vi "execute.vi"(8 "error in (no error)":errorcluster, 9 "ParameterString":string, 10 "ObjectCluster":T1, 11 "AirConditionCommand in":refnum<class "AirConditionCommand.lvclass">) -> (0 "error out":errorcluster, 2 "ObjectCluster Out":T1, 3 "AirConditionCommand out":refnum<class "AirConditionCommand.lvclass">)   [LabVIEW 2013, in "AirConditionCommand.lvclass"]
uses:
  AirConditionCommand.lvclass
  Command.lvclass/ObjectCluster.ctl
  AirCondition.lvclass/AirCondition.lvclass
  RoomLight.lvclass/RoomLight.lvclass
  OutDoorLight.lvclass/OutDoorLight.lvclass
  Television.lvclass/Television.lvclass
  Stereo.lvclass/Stereo.lvclass
  Command.lvclass/Command.lvclass
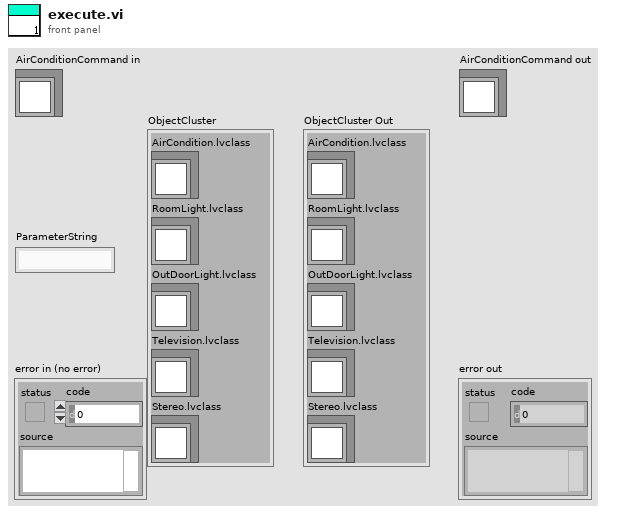
[diagram p1: front panel]
types:
  T1 = typedef "Command.lvclass/ObjectCluster.ctl" = cluster{"AirCondition.lvclass":refnum<class "AirCondition.lvclass">, "RoomLight.lvclass":refnum<class "RoomLight.lvclass">, "OutDoorLight.lvclass":refnum<class "OutDoorLight.lvclass">, "Television.lvclass":refnum<class "Television.lvclass">, "Stereo.lvclass":refnum<class "Stereo.lvclass">}
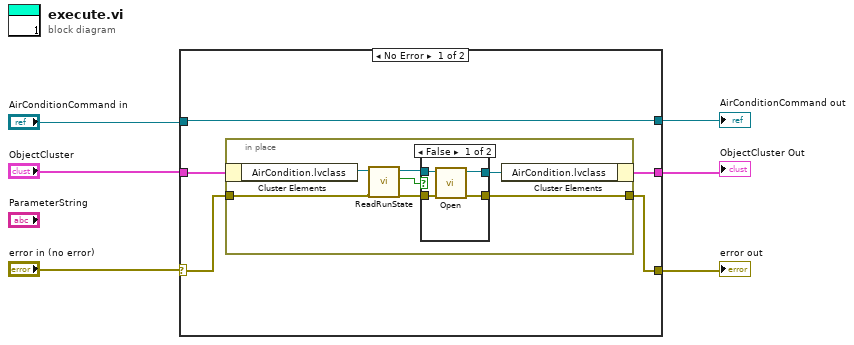
[diagram p0: block diagram]
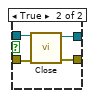
[diagram p2: hidden frame]
diagram:
  n1 = case shown="No Error" "error in (no error)" {
    selector: "error in (no error)" -> [w10 w27]
    tunnel: "ObjectCluster" -> [w11 w28]
    tunnel: "AirConditionCommand in" -> [w7 w29]
    tunnel: [w9 w27] -> w2
    tunnel: [w8 w28] -> w1
    tunnel: [w7 w29] -> w5
    frame No Error {
      n2 = in-place {
        in-place-border: w10 -> [w15]
        in-place-border: [w17] -> w9
        n3 = in-place-cluster #1(w11) -> ("AirCondition.lvclass"=w16:refnum<class "AirCondition.lvclass">)
        n4 = call-dynamic "ReadRunState.vi"("error in (no error)"=w15, "AirCondition in"=w16) -> ("error out"=w14:errorcluster, "RunState"=w12:bool, "AirCondition out"=w13:refnum<class "AirCondition.lvclass">)  [unwired: 7 in]
        n5 = case shown="False" w12 {
          tunnel: w13 -> [w19 w25]
          tunnel: w14 -> [w22 w26]
          tunnel: [w20 w24] -> w18
          tunnel: [w21 w23] -> w17
          frame False {
            n6 = call-dynamic "Open.vi"("error in (no error)"=w22, "AirCondition in"=w19) -> ("error out"=w21:errorcluster, "AirCondition out"=w20:refnum<class "AirCondition.lvclass">)  [unwired: 8 in]
          }
          frame True {
            n7 = call-dynamic "Close.vi"("error in (no error)"=w26, "AirCondition in"=w25) -> ("error out"=w23:errorcluster, "AirCondition out"=w24:refnum<class "AirCondition.lvclass">)  [unwired: 8 in]
          }
        }
        n8 = in-place-cluster #1("AirCondition.lvclass"=w18) -> (w8:T1)
      }
    }
    frame Error {
    }
  }
  "error out" <- w2
  "AirConditionCommand out" <- w5
  "ObjectCluster Out" <- w1
